vi "sgFilter_gyro.vi"() -> ()   [LabVIEW 2011]
uses:
  <vilib>/Analysis/3filter.llb/Savitzky-Golay Filter (DBL).vi
  <vilib>/Analysis/NI_AALBase.lvlib
panel:
  out "Filtered X":dbl[](array[numeric])
  in  "stop":bool
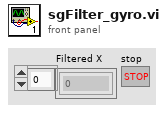
[diagram p1: front panel]
types:
  T1 = typedef "WPI_GyroDevRef.ctl" = cluster{"DevStatus":errorcluster, "Analog Module":T2, "Analog Channel":T3, "Offset":dbl, "Gain (VoltsPerDegree/Second)":dbl}
  T2 = typedef "FPGA_TypedefAnalogModule.ctl" = enum16{"Analog Module 1", "Analog Module 2"}
  T3 = typedef "FPGA_AIChannel.ctl" = enum8{"AI 1", "AI 2", "AI 3", "AI 4", "AI 5", "AI 6", "AI 7", "AI 8", "Invalid"}
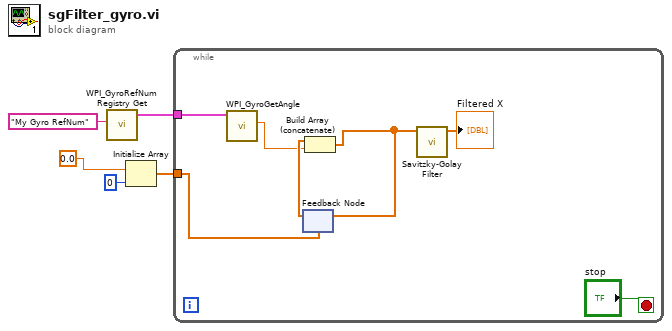
[diagram p0: block diagram]
diagram:
  n1 = call <vilib>:"WPI_GyroRefNum Registry Get.vi"("refnum name"="My Gyro RefNum") -> ("GyroDevRef"=w5:T1)  [unwired: 9 in, 1 out]
  n2 = Initialize Array(0.0, 0 ("dimension size")) -> (w2:dbl[])
  n3 = while {
    tunnel: w5 -> [w12]
    tunnel: w2 -> [w10]
    stop <- "stop" stop-if-true
    n4 = call <vilib>:"WPI_GyroGetAngle.vi"("GyroDevRef"=w12) -> ("Angle"=w8:dbl)  [unwired: 7 in, 3 out]
    n5 = feedback #1(w10) -> (w9:dbl[])
    n6 = Build Array (concatenate)(w9, w8) -> (w7:dbl[])
    n7 = feedback-in #1(w7) -> ()
    n8 = call-poly <vilib>:"Savitzky-Golay Filter.vi"("X"=w7) -> ("Filtered X"=→"Filtered X":dbl[])  [unwired: 9 in, 1 out]
  }
